vi "ReadAuto.vi"(8 "error in":errorcluster) -> (0 "error out":errorcluster)   [LabVIEW 2017]
uses:
  <vilib>/Utility/file.llb/Read Delimited Spreadsheet (string).vi
panel:
  in  "delimiter (,)":string="\t"
  in  "file path (dialog if empty)":path
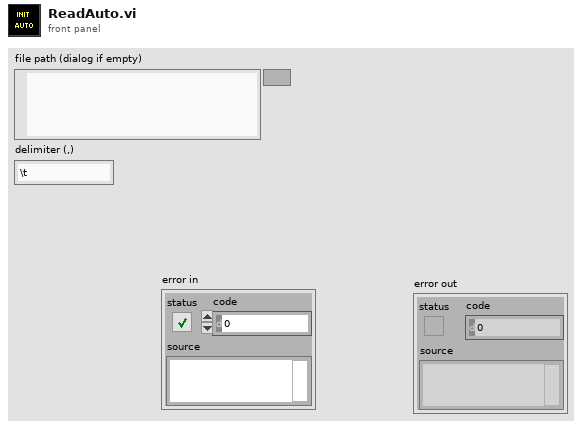
[diagram p1: front panel]
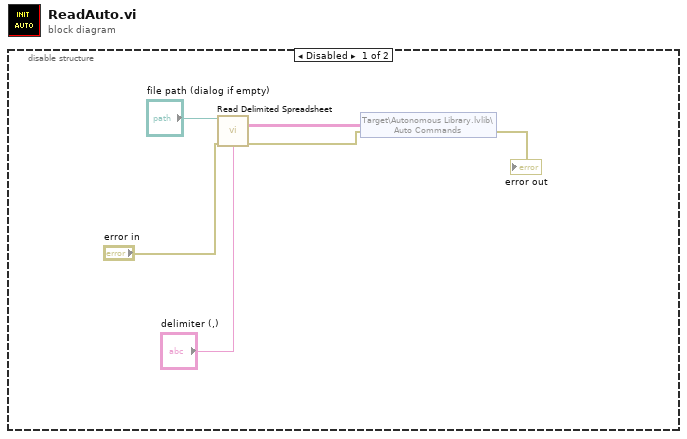
[diagram p0: block diagram]
diagram:
  n1 = disable-structure shown="Disabled" {
    frame Disabled {
      n2 = call-poly <vilib>:"Read Delimited Spreadsheet.vi"("file path (dialog if empty)"="file path (dialog if empty)", "error in (no error)"="error in", "delimiter (\\t)"="delimiter (,)") -> ("all rows"=w3:string[][], "error out"=w2:errorcluster)  [unwired: 7 in, 4 out]
      n3 = shared-variable "Target\\Autonomous Library.lvlib\\Auto Commands"(w3, error in=w2) -> (error out=→"error out":errorcluster)
    }
    frame Enabled {
    }
  }
